vi "Waypoints Generator.vi"(4 "invertPath":bool, 6 "startingPoint":dbl[](array[numeric]), 7 "direction":dbl, 8 "changeDir":bool, 9 "l":dbl, 10 "h":dbl, 11 "numPoints":dbl) -> (3 "grid":dbl[][](array[numeric]))   [LabVIEW 2014]
uses:
  <vilib>/imath/engines/lvmath2/RunTimeEngine/Managers/WorkSpace/UID Generator.vi
  <vilib>/imath/engines/lvmath2/RunTimeEngine/IndexReplace/NIMS M(S,$)=V.vi
  <instcachedir>/0/NIMS M(S,$)=V_8321FD9A786642FB877A2933E8B48D2A.lvgen/NIMS M(S,$)=V_8321FD9A786642FB877A2933E8B48D2A_001.vi
  <vilib>/imathl/engines/lvmath/Functions/Error Handling/Create Error.vi
  <vilib>/imath/engines/lvmath2/RunTimeEngine/CommandStatement/MC_CommandStatement_break.vi
  <vilib>/imath/engines/lvmath2/RunTimeEngine/IndexRead/NIMS M(S,S).vi
  <instcachedir>/0/NIMS M(S,S)_AC51E74150A542F7991B9634C66F3096.lvgen/NIMS M(S,S)_AC51E74150A542F7991B9634C66F3096_000.vi
  <vilib>/imath/engines/lvmath2/RunTimeEngine/IndexReplace/NIMS M(S,S)=S.vi
  <instcachedir>/0/NIMS M(S,S)=S_43446D47E75543269C90719353EB0EB0.lvgen/NIMS M(S,S)=S_43446D47E75543269C90719353EB0EB0_000.vi
  <vilib>/imath/engines/lvmath2/RunTimeEngine/ErrorHandling/NIMS_Create Error From Enums.vi
  <vilib>/imath/engines/lvmath2/RunTimeEngine/CommandStatement/NIMS_CommandStatement_MaskErr.vi
  <vilib>/imath/engines/lvmath2/RunTimeEngine/RangeToken/NIMS_Range.vi
  <instcachedir>/0/NIMS_Range_9BCE657718DF4976A877346C61F22738.lvgen/NIMS_Range_9BCE657718DF4976A877346C61F22738_000.vi
  <vilib>/imath/engines/lvmath2/RunTimeSupport/NIMS_Error if Not Equal.vi
  <instcachedir>/0/NIMS_Error if Not Equal_8A0E9F659B9142D69417CC259581C4FD.lvgen/NIMS_Error if Not Equal_8A0E9F659B9142D69417CC259581C4FD_001.vi
  <vilib>/imath/engines/lvmath2/RunTimeEngine/IndexRead/NIMS M(V,$).vi
  <instcachedir>/0/NIMS M(V,$)_21A5155762F74C04AE4EA67BEE0D3EF5.lvgen/NIMS M(V,$)_21A5155762F74C04AE4EA67BEE0D3EF5_004.vi
  <vilib>/imath/engines/lvmath2/RunTimeEngine/RunTimeType/NIMS_RunTimeType_From StrictType (excl LVString).vi
  <instcachedir>/0/NIMS_RunTimeType_From StrictType (excl LVString)_15A5391EEA9C4AACB9955AC755B83D29.lvgen/NIMS_RunTimeType_From StrictType (excl LVString)_15A5391EEA9C4AACB9955AC755B83D29_000.vi
  <vilib>/imath/engines/lvmath2/RunTimeEngine/LocalVariableDefStatement/MC_LocalVariableDefStatement_Display.vi
  <vilib>/imath/engines/lvmath2/RunTimeEngine/IndexRead/NIMS M($,S).vi
  <instcachedir>/0/NIMS M($,S)_3E5749BBB62E49528D4765A77F1F6D98.lvgen/NIMS M($,S)_3E5749BBB62E49528D4765A77F1F6D98_000.vi
  <vilib>/imath/engines/lvmath2/RunTimeEngine/IndexReplace/NIMS M($,S)=V.vi
  <instcachedir>/0/NIMS M($,S)=V_9A2C45A15D35467AAEE2181FC06185DD.lvgen/NIMS M($,S)=V_9A2C45A15D35467AAEE2181FC06185DD_001.vi
  <vilib>/imath/engines/lvmath2/RunTimeEngine/ArithmeticOperatorToken/NIMS_ArithmeticOperator_multmx.vi
  <instcachedir>/0/NIMS_ArithmeticOperator_multmx_CE3986B82B8C4E94A31593A7EF82383B.lvgen/NIMS_ArithmeticOperator_multmx_CE3986B82B8C4E94A31593A7EF82383B_004.vi
  <vilib>/imath/engines/lvmath2/RunTimeEngine/RangeToken/NIMS_Range_R3 - Float.vi
  <instcachedir>/0/NIMS_Range_R3 - Float_8F02802A7F4A4758B2B43BD6E2032D09.lvgen/NIMS_Range_R3 - Float_8F02802A7F4A4758B2B43BD6E2032D09_000.vi
  <instcachedir>/0/NIMS_Error if Not Equal_8A0E9F659B9142D69417CC259581C4FD.lvgen/NIMS_Error if Not Equal_8A0E9F659B9142D69417CC259581C4FD_000.vi
  <vilib>/imath/engines/lvmath2/RunTimeEngine/IndexRead/NIMS M(S,$).vi
  <instcachedir>/0/NIMS M(S,$)_F24F360562DE41D8BE234322A2E15C65.lvgen/NIMS M(S,$)_F24F360562DE41D8BE234322A2E15C65_000.vi
  <vilib>/imath/engines/lvmath2/RunTimeEngine/IndexRead/NIMS V(R2).vi
  <instcachedir>/0/NIMS V(R2)_C76619605A0E4E9F8B2FA9389712AC47.lvgen/NIMS V(R2)_C76619605A0E4E9F8B2FA9389712AC47_000.vi
  <vilib>/imath/engines/lvmath2/RunTimeEngine/ArithmeticOperatorToken/NIMS_ArithmeticOperator_plus.vi
  <instcachedir>/0/NIMS_ArithmeticOperator_plus_48D6EAACA5D645B09F7EC9C016C2DEA8.lvgen/NIMS_ArithmeticOperator_plus_48D6EAACA5D645B09F7EC9C016C2DEA8_004.vi
  <instcachedir>/0/NIMS M(S,$)=V_8321FD9A786642FB877A2933E8B48D2A.lvgen/NIMS M(S,$)=V_8321FD9A786642FB877A2933E8B48D2A_000.vi
  <vilib>/imath/engines/lvmath2/RunTimeEngine/IndexRead/NIMS V(S).vi
  <instcachedir>/0/NIMS V(S)_0488751826AF41519A22953C041130DC.lvgen/NIMS V(S)_0488751826AF41519A22953C041130DC_000.vi
  <vilib>/imath/engines/lvmath2/RunTimeEngine/IndexReplace/NIMS M($,S)=S.vi
  <instcachedir>/0/NIMS M($,S)=S_2513D75E6F1349BCA18E26BA96FD1C01.lvgen/NIMS M($,S)=S_2513D75E6F1349BCA18E26BA96FD1C01_000.vi
  <vilib>/imath/engines/lvmath2/RunTimeEngine/BuiltInFunctions/length/NIMS_length(GV).vi
  <instcachedir>/0/NIMS_length(GV)_08A3D13377FD4E4B96F5795FBF3698FA.lvgen/NIMS_length(GV)_08A3D13377FD4E4B96F5795FBF3698FA_000.vi
  <vilib>/imath/engines/lvmath2/RunTimeEngine/RangeToken/NIMS_Range_R3 - Integer.vi
  <instcachedir>/0/NIMS_Range_R3 - Integer_66B9031982364693905FDE422E56E490.lvgen/NIMS_Range_R3 - Integer_66B9031982364693905FDE422E56E490_000.vi
  <vilib>/imath/engines/lvmath2/RunTimeEngine/IndexRead/NIMS M(S,R2).vi
  <instcachedir>/0/NIMS M(S,R2)_45730E4D0DB74D118F715F4F99DCE4D7.lvgen/NIMS M(S,R2)_45730E4D0DB74D118F715F4F99DCE4D7_000.vi
  <vilib>/imath/engines/lvmath2/RunTimeEngine/IndexReplace/NIMS M(S,R2)=V.vi
  <instcachedir>/0/NIMS M(S,R2)=V_74719D1886FD41299CC34F2C1799E6B7.lvgen/NIMS M(S,R2)=V_74719D1886FD41299CC34F2C1799E6B7_000.vi
  <vilib>/imath/engines/lvmath2/RunTimeEngine/Managers/SymbolTable/Clear UID.vi
  <vilib>/imath/engines/lvmath2/RunTimeEngine/NodeEndStatement/NIMS_NodeEndStatement_Output.vi
  <instcachedir>/0/NIMS_NodeEndStatement_Output_53EC0D466D134D7ABD903AC30B43404B.lvgen/NIMS_NodeEndStatement_Output_53EC0D466D134D7ABD903AC30B43404B_002.vi
  <vilib>/imath/engines/lvmath2/RunTimeEngine/ErrorHandling/NIMS_Finalize Error.vi
  <vilib>/imath/engines/lvmath2/RunTimeEngine/Managers/SymbolTable/NIMS_WorkSpace.lvlib
panel:
  in  "offset":dbl
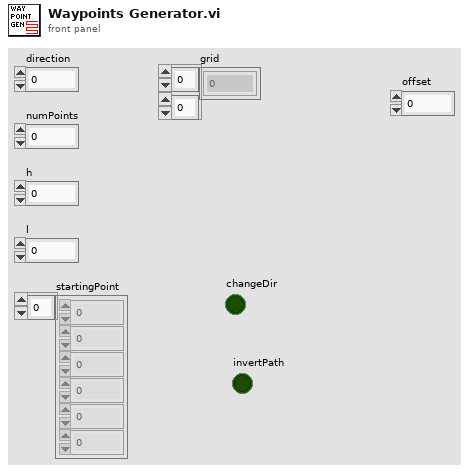
[diagram p1: front panel]
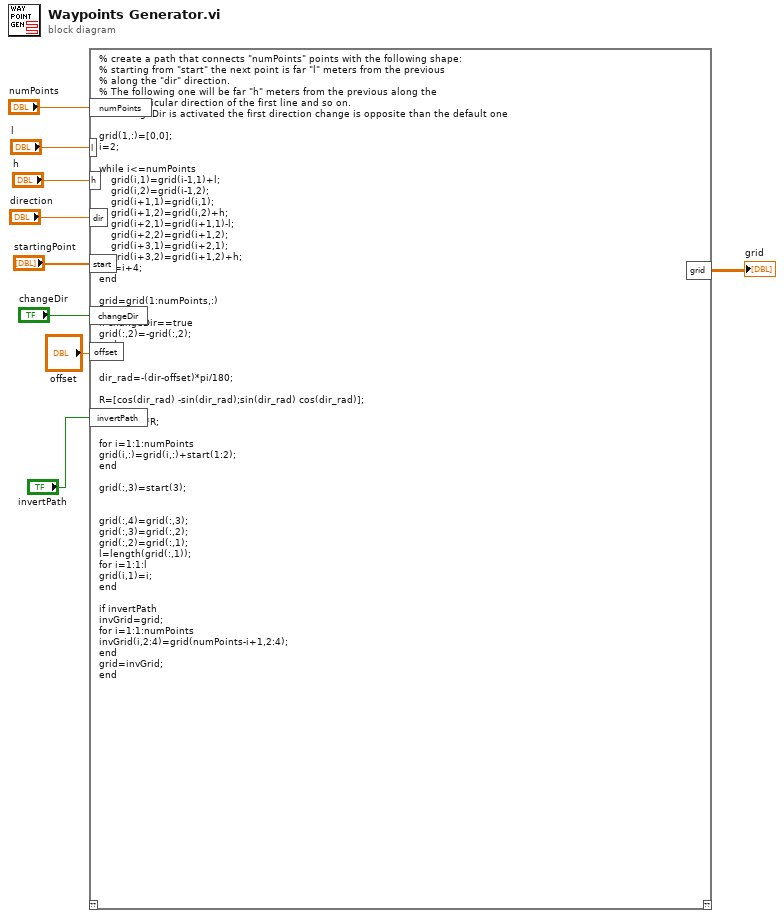
[diagram p0: block diagram]
diagram:
  n1 = mathscript code="% create a path that connects \"numPoints\" points with the following shape:\n% starting from \"start\" the next point is far \"l\" meters from the previous\n% along the \"dir\" direction. \n% The following one will be far \"h\" meters from the previous along the \n% perpendicular direction of the first line and so on.\n%If changeDir is activated the first direction change is opposite than the default one\n\ngrid(1,:)=[0,0];\ni=2;\n\nwhile i<=numPoints \n    grid(i,1)=grid(i-1,1)+l;\n    grid(i,2)=grid(i-1,2);\n    grid(i+1,1)=grid(i,1);\n    grid(i+1,2)=grid(i,2)+h;\n    grid(i+2,1)=grid(i+1,1)-l;\n    grid(i+2,2)=grid(i+1,2);\n    grid(i+3,1)=grid(i+2,1);\n    grid(i+3,2)=grid(i+1,2)+h;\n    i=i+4;\nend\n\ngrid=grid(1:numPoints,:)\n\nif changeDir==true\ngrid(:,2)=-grid(:,2);\nend\n\n\ndir_rad=-(dir-offset)*pi/180;\n\nR=[cos(dir_rad) -sin(dir_rad);sin(dir_rad) cos(dir_rad)];\n\ngrid=grid*R;\n\nfor i=1:1:numPoints\ngrid(i,:)=grid(i,:)+start(1:2);\nend\n\ngrid(:,3)=start(3);\n\n\ngrid(:,4)=grid(:,3);\ngrid(:,3)=grid(:,2);\ngrid(:,2)=grid(:,1);\nl=length(grid(:,1));\nfor i=1:1:l\ngrid(i,1)=i;\nend\n\nif invertPath\ninvGrid=grid;\nfor i=1:1:numPoints\ninvGrid(i,2:4)=grid(numPoints-i+1,2:4);\nend\ngrid=invGrid;\nend"("numPoints"="numPoints", "l"="l", "h"="h", "dir"="direction", "start"="startingPoint", "changeDir"="changeDir", "offset"="offset", "invertPath"="invertPath") -> ("grid"=→"grid":dbl[][])  [unwired: 1 in, 1 out]
